vi "Stop-Set.vi"(8 "error in (no error)":errorcluster, 10 "Reason":string, 11 "StopSignal Name(\"\" to use topmostVI)":string) -> (0 "error out":errorcluster)   [LabVIEW 2017, in "StopSignal.lvlib"]
uses:
  StopSignal.lvlib
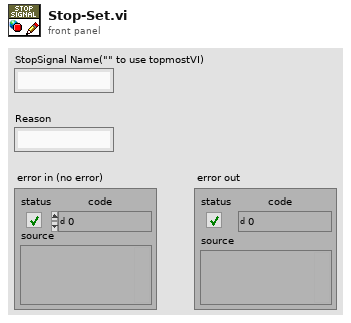
[diagram p1: front panel]
types:
  T1 = typedef "StopSignal.lvlib/StopSignal.ctl" = refnum<k1>
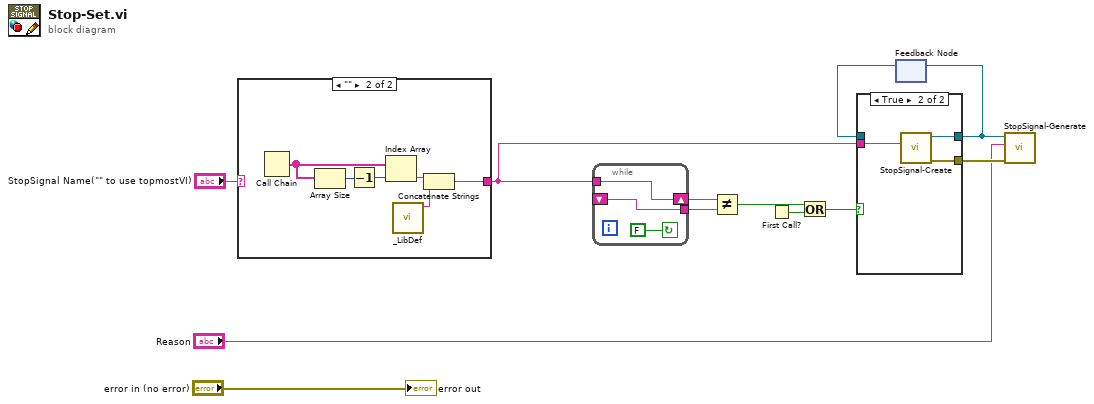
[diagram p0: block diagram]
diagram:
  n1 = case shown="\"\"" "StopSignal Name(\"\" to use topmostVI)" {
    selector: "StopSignal Name(\"\" to use topmostVI)" -> [w13 _]
    tunnel: [w13 w14] -> w7
    frame "False", Default {
    }
    frame "" {
      n2 = Call Chain() -> (call chain=w17:string[])
      n3 = Array Size(array=w17) -> (size(s)=w19:i32)
      n4 = Decrement(x=w19) -> (x-1=w18:i32)
      n5 = Index Array(array=w17, index=w18) -> (element=w16:string)
      n6 = call "_LibDef.vi"() -> ("LIBNAME"=w15:string)  [unwired: 11 in]
      n7 = Concatenate Strings(w16, w15) -> (w14:string)
    }
  }
  n8 = while {
    shift-right: [w22] -> w2
    shift-left: _ -> [w21]
    tunnel: w7 -> [w22]
    tunnel: [w21] -> w3
    stop <- FALSE continue-if-true
  }
  n9 = Not Equal?(x=w2, y=w3) -> (x != y?=w1:bool)
  n10 = First Call?() -> (First Call?: T/F=w10:bool)
  n11 = Or(x=w1, y=w10) -> (x .or. y?=w9:bool)
  n12 = feedback #1() -> (w8:T1)  [unwired: 1 in]
  n13 = case shown="True" w9 {
    tunnel: [_ w26] -> w12
    tunnel: [w23 w25] -> w11
    tunnel: w8 -> [w23 _]
    tunnel: w7 -> [_ w24]
    frame False {
    }
    frame True {
      n14 = call "StopSignal-Create.vi"("name(\"\")"=w24) -> ("error out"=w26:errorcluster, "StopSignal"=w25:T1)  [unwired: 9 in]
    }
  }
  n15 = feedback-in #1(w11) -> ()
  n16 = call "StopSignal-Generate.vi"("error in (no error)"=w12, "reason(\"\")"="Reason", "StopSignal"=w11) -> ()  [unwired: 7 in, 2 out]
  "error out" <- "error in (no error)"
